vi "Scheme.Update Image (Multiple).vi"(6 "Replace Image":path[](array[path]), 8 "error in":errorcluster, 9 "New Color":u32[](array[colorbox]), 10 "New Control":path, 11 "Material-Scheme.lvclass":refnum<class "Material-Scheme.lvclass">) -> (0 "error out":errorcluster, 3 "Material-Scheme.lvclass out":refnum<class "Material-Scheme.lvclass">, 4 "image":path)   [LabVIEW 2021, in "TSC Material Theme.lvlib" / "Material-Scheme.lvclass"]
doc: "Update the image on a multi-image button.\n\n<b>Code Developed By:</b> +\nDaniel Coons +\nTechnology Service Corporation +\nwww.tsc.com/atcs"
uses:
  Material-Scheme.lvclass
  private/Insert TSC tEXt Chunk.vi
  Material SubVIs/Material SubVIs.lvlib
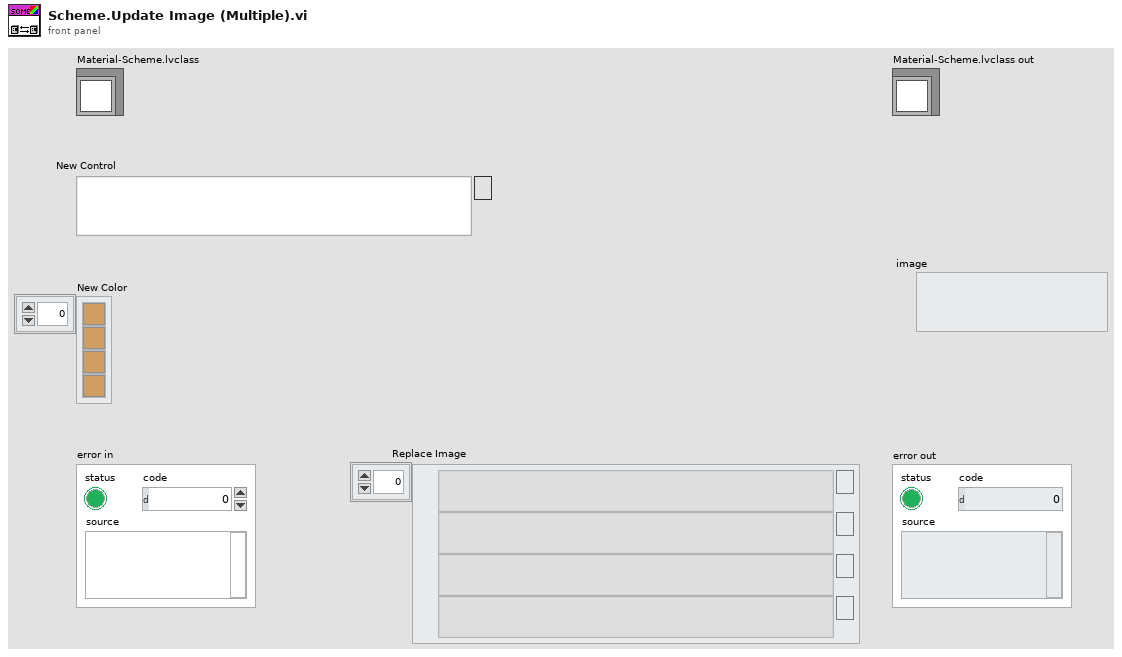
[diagram p1: front panel]
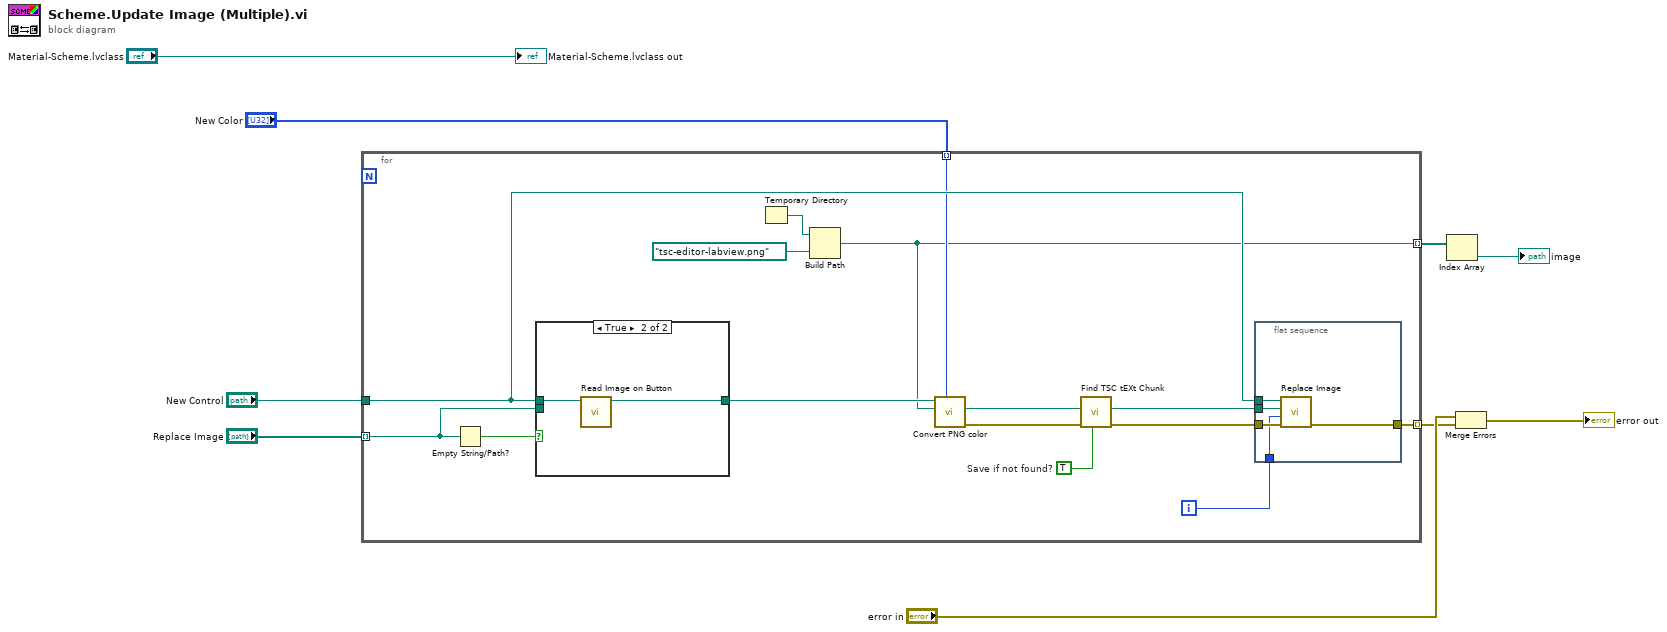
[diagram p0: block diagram]
diagram:
  n1 = for {
    tunnel: "New Control" -> [w23]
    tunnel: "Replace Image" -> [w22] mode=indexing
    tunnel: [w21] -> w4 mode=indexing
    tunnel: "New Color" -> [w17] mode=indexing
    tunnel: [w11] -> w2 mode=indexing
    i -> [w10]
    w13 = TRUE  # Save if not found?
    n2 = Empty String/Path?(string/path=w22) -> (empty?=w24:bool)
    n3 = case shown="True" w24 {
      tunnel: [w30 w32] -> w20
      tunnel: w23 -> [_ w31]
      tunnel: w22 -> [w30 _]
      frame False {
      }
      frame True {
        n4 = call "Read Image on Button.vi"("File with Button"=w31) -> ("png file out"=w32:path)  [unwired: 9 in, 1 out]
      }
    }
    n5 = Temporary Directory() -> (w19:path)
    n6 = Build Path(base path=w19, name or relative path=path "tsc-editor-labview.png") -> (appended path=w11:path)
    n7 = call "Convert PNG color.vi"("New Color"=w17, "new file"=w11, "orig file"=w20) -> ("error out"=w16:errorcluster, "new file out"=w14:path)  [unwired: 6 in, 1 out]
    n8 = call "Find TSC tEXt Chunk.vi"("Save if not found?"=w13, "error in"=w16, "file path (use dialog)"=w14) -> ("error out"=w15:errorcluster, "file path dup"=w12:path)  [unwired: 6 in, 1 out]
    n9 = flat-sequence {
      tunnel: w23 -> [w29]
      tunnel: w15 -> [w28]
      tunnel: [w27] -> w21
      tunnel: w12 -> [w26]
      tunnel: w10 -> [w25]
      frame #0 {
        n10 = call "Replace Image.vi"("error in"=w28, "image item"=w25, "PNG Image File"=w26, "LabVIEW File with Button"=w29) -> ("error out"=w27:errorcluster)  [unwired: 6 in, 1 out]
      }
    }
  }
  n11 = Index Array(array=w2) -> (element=→"image":path)  [unwired: 1 in]
  n12 = Merge Errors("error in", w4) -> (→"error out":errorcluster)
  "Material-Scheme.lvclass out" <- "Material-Scheme.lvclass"
